vi "Process IMAQ Image (Webcam).vi"() -> ()   [LabVIEW 2020]
uses:
  <vilib>/userDefined/High Color/IMAQdx.ctl
  <vilib>/vision/driver/IMAQdx.llb/IMAQdx Buffer Number Mode.ctl
  6d5f1638-640c-4e20-b011-0cee3ae60b95.vi
  688a6956-cd2d-4b8a-a8be-e172edc5432f.vi
  45820c2d-b3f1-45d5-9983-17417cdda85c.vi
  G-Embedded-Python-Interpreter-Toolkit/Null Py Object Refnum.vi
  6d5f1638-640c-4e20-b011-0cee3ae60b95.vi/96ddca92-7bbf-40e2-a1a5-d32f291eb6af.vi
  G-Embedded-Python-Interpreter-Toolkit-IMAQ/IMAQ to Py Object.vi/22f05568-5bba-4402-9e98-aca160827363.vi
  688a6956-cd2d-4b8a-a8be-e172edc5432f.vi/6c7a13f1-33d3-431d-8188-904cac5422b3.vi
  45820c2d-b3f1-45d5-9983-17417cdda85c.vi/6c7a13f1-33d3-431d-8188-904cac5422b3.vi
  G-Embedded-Python-Interpreter-Toolkit/Python Object Reference to Pointer Sized Ref.vi
  G-Embedded-Python-Interpreter-Toolkit/Pointer Sized Ref to Python Object Reference.vi
  G-Embedded-Python-Interpreter-Toolkit/Merge Call Library Errors.vi
  G-Embedded-Python-Interpreter-Toolkit/Generate Argument Type Info.vi
  G-Embedded-Python-Interpreter-Toolkit/Create Py Object IMAQ Image.vi
  G-Embedded-Python-Interpreter-Toolkit/G-Embedded-Python-Interpreter-Toolkit.lvlib
  G-Embedded-Python-Interpreter-Toolkit-IMAQ/G-Embedded-Python-Interpreter-Toolkit-IMAQ.lvlib
  <vilib>/vision/driver/NI_Vision_Acquisition_Software.lvlib
panel:
  in  "stop":bool
  out "Image":T1(plugin-control)
  in  "Session In":T2="cam0"
  out "Print Ouptut":string
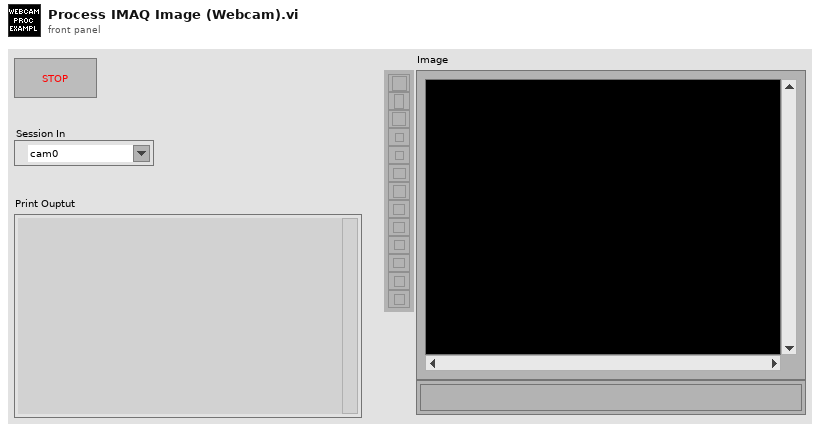
[diagram p1: front panel]
types:
  T1 = typedef "IMAQ Image.ctl" = refnum<image>
  T2 = typedef "IMAQdx.ctl" = refnum<k21>
  T3 = typedef "Image Type" = u32
  T4 = typedef "G-Embedded-Python-Interpreter-Toolkit.lvlib/Python Object Reference.ctl" = refnum<k1>
  T5 = typedef "NI_Vision_Acquisition_Software.lvlib/IMAQdx Buffer Number Mode.ctl" = enum32{"Next", "Last", "Buffer Number", "Every", "Last New"}
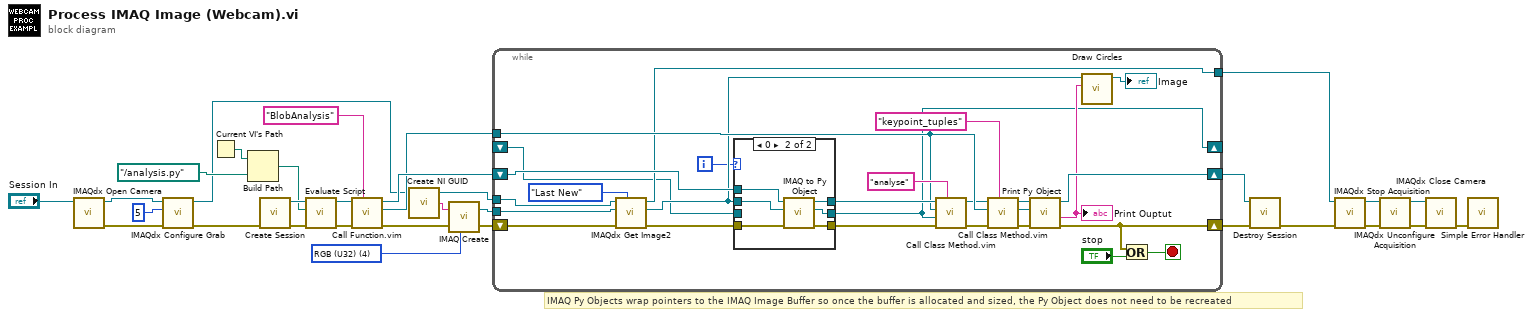
[diagram p0: block diagram]
diagram:
  w23 = T3 4 items=["Grayscale (U8)", "Grayscale (I16)", "Grayscale (SGL)", "Complex (CSG)", "RGB (U32)", "HSL (U32)", "RGB (U64)", "Grayscale (U16)"] ("Image Type")
  # "IMAQ Py Objects wrap pointers to the IMAQ Image Buffer so once the buffer is allocated and sized, the Py Object does not need to be recreated"
  n1 = call <vilib>:"IMAQdx Open Camera.vi"("Session In"="Session In") -> ("error out"=w11:errorcluster, "Session Out"=w12:T2)  [unwired: 9 in]
  n2 = call <vilib>:"IMAQdx Configure Grab.vi"("error in"=w11, "Number of Buffers"=u32 5, "Session In"=w12) -> ("error out"=w2:errorcluster, "Session Out"=w9:T2)  [unwired: 7 in]
  n3 = Current VI's Path() -> (path=w21:path)
  n4 = Build Path(base path=w21, name or relative path=path "../analysis.py") -> (appended path=w27:path)
  n5 = call "Create Session.vi"("error in (no error)"=w2) -> ("error out"=w30:errorcluster, "Session Handle"=w29:refnum<data-value>)  [unwired: 9 in]
  n6 = call "Evaluate Script.vi"("error in (no error)"=w30, "Script File Path"=w27, "Session Handle in"=w29) -> ("error out"=w24:errorcluster, "Session Handle out"=w25:refnum<data-value>)  [unwired: 7 in]
  n7 = call "Call Function.vim"("Function Name"="BlobAnalysis", "error in (no error)"=w24, "Data Value Reference in"=w25) -> ("error out"=w22:errorcluster, "Returned Python Object Refnum"=w18:T4, "Data Value Reference out"=w20:refnum<data-value>)  [unwired: 6 in]
  n8 = call <vilib>:"Create NI GUID.vi"() -> ("NI GUID"=w19:string)
  n9 = call "IMAQ Create"("Image Name"=w19, "Image Type"=w23, "error in (no error)"=w22) -> ("New Image"=w14:T1, "error out"=w13:errorcluster)  [unwired: 2 in]
  n10 = while {
    tunnel: w18 -> [w52]
    tunnel: w14 -> [w45]
    shift-right: [w46] -> w17
    shift-left: w20 -> [w56]
    shift-right: [w40] -> w16
    shift-left: w13 -> [w44]
    tunnel: w9 -> [w38]
    tunnel: [w37] -> w4
    shift-right: [w32] -> _
    shift-left: _ -> [w31]
    i -> [w33]
    stop <- w41 stop-if-true
    n11 = call <vilib>:"IMAQdx Get Image2.vi"("Buffer Number Mode (Next)"=IMAQdx_Buffer_Number_Mode."Last New", "error in"=w44, "Image In"=w45, "Session In"=w38) -> ("error out"=w43:errorcluster, "Image Out"=w36:T1, "Session Out"=w37:T2)  [unwired: 4 in, 1 out]
    n12 = case shown="0" w33 {
      tunnel: w56 -> [w58 w66]
      tunnel: [w58 w65] -> w55
      tunnel: [w60 w64] -> w54
      tunnel: [w59 w63] -> w32
      tunnel: w43 -> [w60 w62]
      tunnel: w36 -> [_ w61]
      tunnel: w31 -> [w59 _]
      frame Default {
      }
      frame 0 {
        n13 = call "IMAQ to Py Object.vi"("error in (no error)"=w62, "Image In"=w61, "Session Handle in"=w66) -> ("error out"=w64:errorcluster, "Python Object Refnum"=w63:T4, "Session Handle out"=w65:refnum<data-value>)  [unwired: 6 in]
      }
    }
    n14 = call "Call Class Method.vim"("Function Name"="analyse", "error in (no error)"=w54, "Arguments in (Default - Empty)"=w32, "Class Instance"=w52, "Data Value Reference in"=w55) -> ("error out"=w53:errorcluster, "Data Value Reference out"=w48:refnum<data-value>)  [unwired: 4 in, 1 out]
    n15 = call "Call Class Method.vim"("Function Name"="keypoint_tuples", "error in (no error)"=w53, "Class Instance"=w52, "Data Value Reference in"=w48) -> ("error out"=w51:errorcluster, "Returned Python Object Refnum"=w49:T4, "Data Value Reference out"=w47:refnum<data-value>)  [unwired: 5 in]
    n16 = call "Print Py Object.vi"("error in (no error)"=w51, "Python Object Refnum in"=w49, "Session Handle in"=w47) -> ("error out"=w40:errorcluster, "Print Ouptut"=w34:string, "Session Handle out"=w46:refnum<data-value>)  [unwired: 5 in, 1 out]
    "Print Ouptut" <- w34
    n17 = call "Draw Circles.vi"("Print Ouptut"=w34, "Refnum in"=w36) -> ("Refnum out"=→"Image":T1)  [unwired: 9 in]
    n18 = Or(x=w40, y="stop") -> (x .or. y?=w41:bool)
  }
  n19 = call "Destroy Session.vi"("error in (no error)"=w16, "Session Handle"=w17) -> ("error out"=w1:errorcluster)  [unwired: 9 in]
  n20 = call <vilib>:"IMAQdx Stop Acquisition.vi"("error in"=w1, "Session In"=w4) -> ("error out"=w8:errorcluster, "Session Out"=w7:T2)  [unwired: 8 out]
  n21 = call <vilib>:"IMAQdx Unconfigure Acquisition.vi"("error in"=w8, "Session In"=w7) -> ("error out"=w5:errorcluster, "Session Out"=w6:T2)  [unwired: 8 out]
  n22 = call <vilib>:"IMAQdx Close Camera.vi"("error in"=w5, "Session In"=w6) -> ("error out"=w3:errorcluster)  [unwired: 9 out]
  n23 = call <vilib>:"Simple Error Handler.vi"("error in (no error)"=w3) -> ()  [unwired: 4 in, 5 out]
